vi "1D Array of VArrays to MultiD Array.vi"(8 "error in (no error)":errorcluster, 9 "Element Type":variant, 10 "Array of VArrays":variant[](array[variant]), 11 "Deserializer in":refnum<class "JSON Deserializer.lvclass">) -> (0 "error out":errorcluster, 2 "MultiD Array":variant, 3 "Deserializer out":refnum<class "JSON Deserializer.lvclass">)   [LabVIEW 2019, in "JKI JSON Serialization.lvlib" / "JSON Deserializer.lvclass"]
doc: "JKI JSON 1.1.10.37\nTomi Maila - JKI\nCopyright (c) 2017, JKI"
uses:
  JSON Deserializer.lvclass
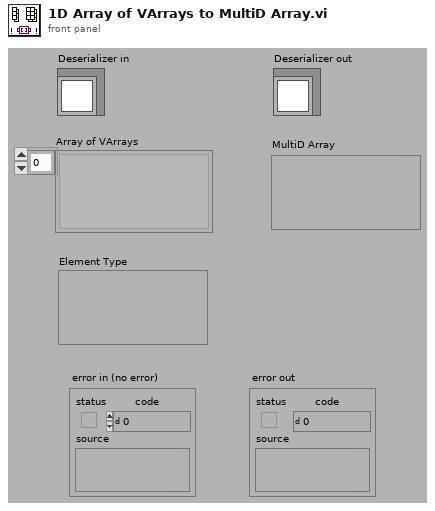
[diagram p1: front panel]
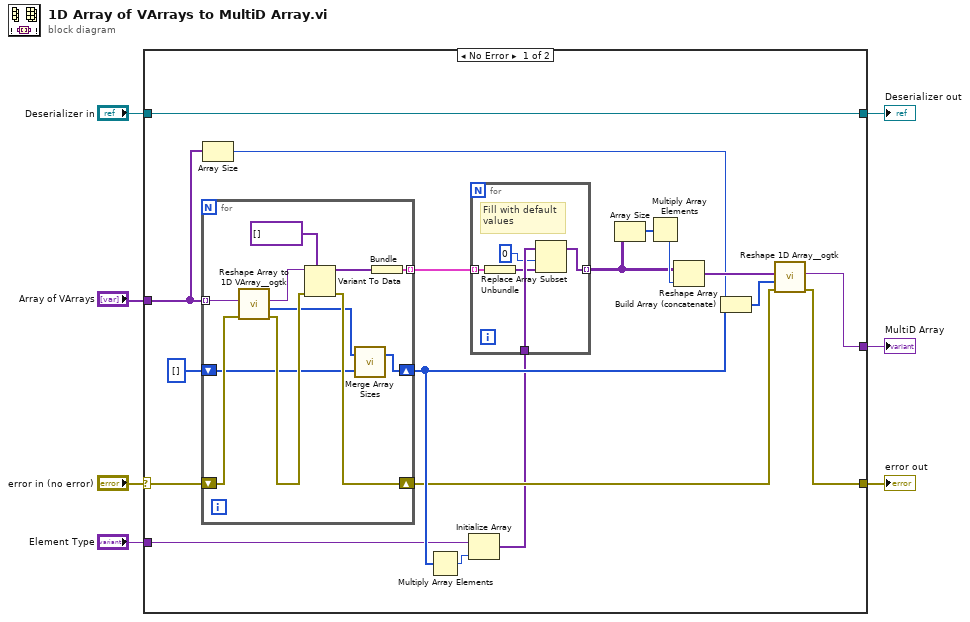
[diagram p0: block diagram]
diagram:
  n1 = case shown="No Error" "error in (no error)" {
    selector: "error in (no error)" -> [w25 w43]
    tunnel: [w20 w43] -> w7
    tunnel: [w17 _] -> w4
    tunnel: "Array of VArrays" -> [w24 _]
    tunnel: "Element Type" -> [w11 _]
    tunnel: "Deserializer in" -> [w8 w42]
    tunnel: [w8 w42] -> w1
    frame No Error {
      n2 = for {
        tunnel: w24 -> [w41] mode=indexing
        shift-right: [w37] -> w12
        shift-left: w25 -> [w40]
        tunnel: [w31] -> w15 mode=indexing
        shift-right: [w33] -> w13
        shift-left: i32[] [] -> [w34]
        n3 = call "Reshape Array to 1D VArray__ogtk.vi"("error in (no error)"=w40, "MultiD Array"=w41) -> ("error out"=w38:errorcluster, "Size(s)"=w32:u32[], "1D VArray"=w39:variant)  [unwired: 7 in]
        n4 = Variant To Data(error in=w38, type=variant[] [], Variant=w39) -> (data=w35:variant[], error out=w37:errorcluster)
        n5 = call "Merge Array Sizes.vi"("Sizes 2"=w34, "Sizes"=w32) -> ("Sizes out"=w33:i32[])  [unwired: 1 in]
        n6 = Bundle(w35) -> (w31:cluster{variant[]})  [unwired: 1 in]
      }
      n7 = Array Size(array=w24) -> (size(s)=w19:i32)
      n8 = Multiply Array Elements(1:w13) -> (0:w10:i32)
      n9 = Initialize Array(w11, w10) -> (w9:variant[])
      n10 = for {
        tunnel: w15 -> [w30] mode=indexing
        tunnel: [w29] -> w14 mode=indexing
        tunnel: w9 -> [w28]
        # "Fill with default\nvalues"
        n11 = Unbundle(w30) -> (w27:variant[])
        n12 = Replace Array Subset(array=w28, new element=w27, index=0) -> (w29:variant[])
      }
      n13 = Array Size(array=w14) -> (size(s)=w23:i32[])
      n14 = Multiply Array Elements(1:w23) -> (0:w22:i32)
      n15 = Reshape Array(w14, w22) -> (w21:variant[])
      n16 = Build Array (concatenate)(w19, w13) -> (w18:i32[])
      n17 = call "Reshape 1D Array__ogtk.vi"("error in (no error)"=w12, "Size(s)"=w18, "1D Array"=w21) -> ("error out"=w20:errorcluster, "Reshaped VArray"=w17:variant)  [unwired: 7 in]
    }
    frame Error {
    }
  }
  "error out" <- w7
  "MultiD Array" <- w4
  "Deserializer out" <- w1
